vi "pathplan.vi"() -> ()   [LabVIEW 2016]
panel:
  out "全场定位错误输出":errorcluster caption="错误输出"
  in  "全场定位串口":refnum<visa-resource-name>="ASRL4::INSTR" caption="全场定位模块"
  out "是否跑完规划路径":bool
  in  "speed_max":dbl[](array[numeric])
  out "路径规划数据写入缓冲区":string
  in  "发送写入":refnum<visa-resource-name>
  in  "车宽的一半":dbl=200.0
  in  "err":dbl[](array[numeric])
  in  "数据发送停止开关":bool
  out "起点监视":sgl[](array[numeric])
  out "全场定位缓冲区监视器":string
  in  "目标位置":dbl[](array[numeric])
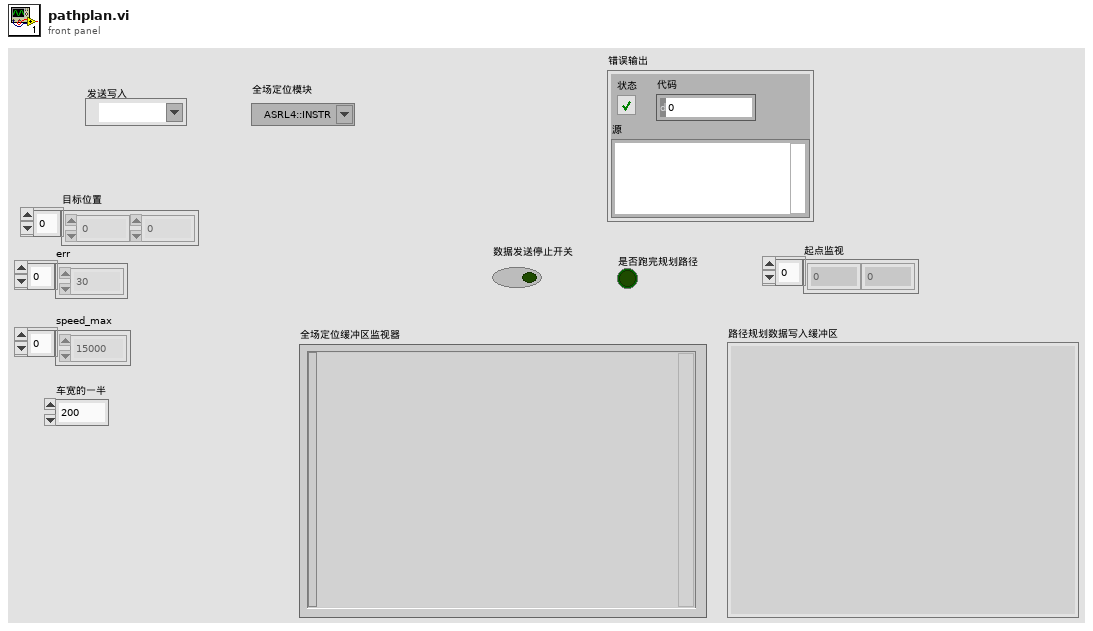
[diagram p1: front panel]
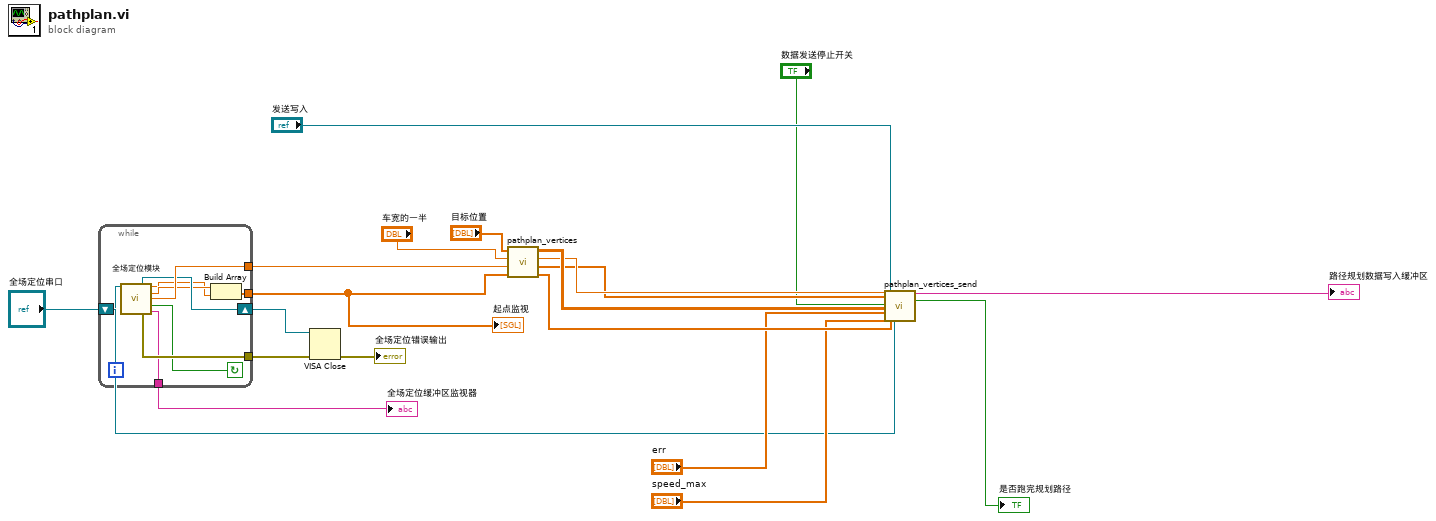
[diagram p0: block diagram]
diagram:
  n1 = while {
    tunnel: [w28] -> w18
    tunnel: [w26] -> w4
    tunnel: [w25] -> w3
    tunnel: [w24] -> w2
    shift-right: [w23] -> w1
    shift-left: "全场定位串口" -> [w27]
    stop <- w22 continue-if-true
    n2 = call "全场定位模块.vi"("VISA resource name"=w27) -> ("VISA资源名称输出"=w23:refnum<visa-resource-name>, "y"=w20:sgl, "x"=w21:sgl, "Zangle"=w24:sgl, "pd"=w22:bool, "错误输出2"=w26:errorcluster, "缓冲区监视器"=w25:string)  [unwired: 8 in]
    n3 = Build Array(w21, w20) -> (w28:sgl[])
  }
  "全场定位缓冲区监视器" <- w3
  "起点监视" <- w18
  n4 = VISA Close(VISA resource name=w1, error in (no error)=w4) -> (error out=→"全场定位错误输出":errorcluster)
  n5 = call "pathplan_vertices.vi"("终点"="目标位置", "车宽的一半"="车宽的一半", "z_angle"=w2, "起点"=w18) -> ("vertices"=w12:dbl[][], "distance_all"=w11:dbl, "angle_all"=w10:dbl[], "distance_send_speed"=w9:dbl[])  [unwired: 3 in]
  n6 = call "pathplan_vertices_send.vi"("distance_all"=w11, "angle_all"=w10, "数据发送停止开关"="数据发送停止开关", "vertices"=w12, "err"="err", "speed_max"="speed_max", "写入串口"="发送写入", "distance_send_speed"=w9, "全场定位串口"="全场定位串口") -> ("路径规划数据写入缓冲区"=→"路径规划数据写入缓冲区":string, "stop_all"=→"是否跑完规划路径":bool)  [unwired: 17 in]
